vi "Get Status.vi"(6 "timeout (ms)":i32=5000, 8 "error in":errorcluster, 11 "gRPC ID":T10) -> (0 "error out":errorcluster, 2 "Node Status":T1 {"Monitor Doubles"."4" format="%#_9g"; "Monitor Doubles"."3" format="%#_9g"; "Monitor Doubles"."2" format="%#_9g"; "Monitor Doubles"."1" format="%#_9g"}, 3 "gRPC ID out":T10)   [LabVIEW 2021, in "CoreGrpcClientWrapper.lvlib"]
uses:
  CoreGrpcClientWrapper.lvlib
  <vilib>/gRPC/LabVIEW gRPC Library/Shared/grpcId.ctl
  CIFTemplateCommon/Typedef/Plugin Status.ctl
  CIFTemplateCommon/Typedef/Plugin State.ctl
  CIFTemplateCommon/Typedef/Timing Statistics.ctl
  CIFTemplateCommon/Typedef/Timing Stats Base.ctl
  CIFTemplateCommon/Typedef/FIFO Statistics.ctl
  CIFTemplateCommon/Typedef/Simple Error.ctl
  CIFTemplateCommon/Typedef/Monitor Doubles.ctl
  CIFTemplateCommon/Typedef/Monitor U64.ctl
  CIFTemplateCommon/Typedef/Monitor I64.ctl
  CIF_Plugin_Core_client/CIF_Plugin_Core_client.lvlib
  CIFTemplateCommon/CIFTemplateCommon.lvlib
  <vilib>/gRPC/LabVIEW gRPC Library/grpc-lvsupport-release.lvlib
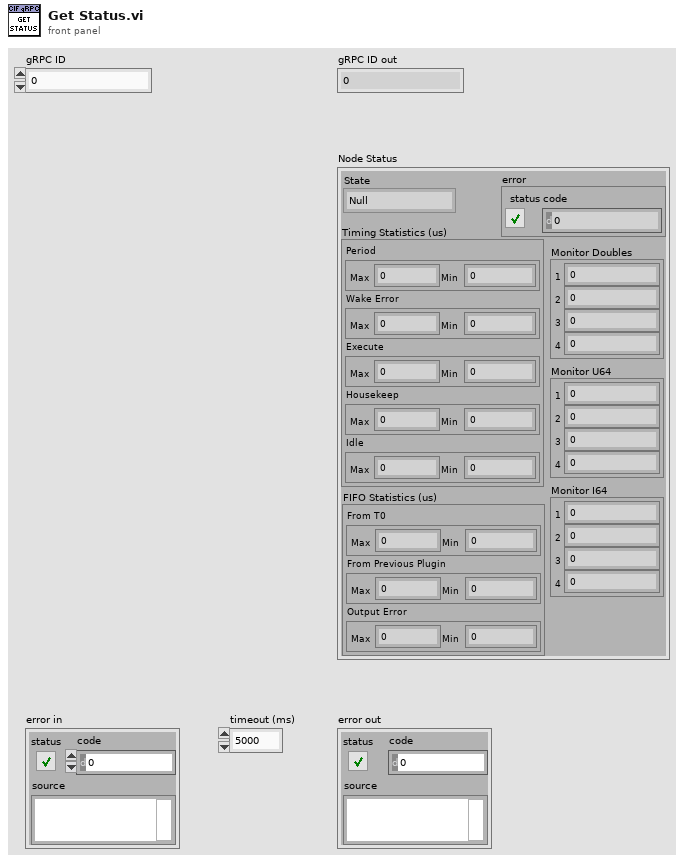
[diagram p1: front panel]
types:
  T1 = typedef "CIFTemplateCommon.lvlib/Plugin Status.ctl" = cluster{"State":T2, "Timing Statistics (us)":T3, "FIFO Statistics (us)":T5, "error":T6, "Monitor Doubles":T7, "Monitor U64":T8, "Monitor I64":T9}
  T2 = typedef "CIFTemplateCommon.lvlib/Plugin State.ctl" = enum32{"Null", "Creating", "Listening", "Running", "CleaningUp", "Destroying"}
  T3 = typedef "CIFTemplateCommon.lvlib/Timing Statistics.ctl" = cluster{"Period":T4, "Wake Error":T4, "Execute":T4, "Housekeep":T4, "Idle":T4}
  T4 = typedef "CIFTemplateCommon.lvlib/Timing Stats Base.ctl" = cluster{"Max":i32, "Min":i32}
  T5 = typedef "CIFTemplateCommon.lvlib/FIFO Statistics.ctl" = cluster{"From T0":T4, "From Previous Plugin":T4, "Output Error":T4}
  T6 = typedef "CIFTemplateCommon.lvlib/Simple Error.ctl" = cluster{"status":bool, "code":i32}
  T7 = typedef "CIFTemplateCommon.lvlib/Monitor Doubles.ctl" = cluster{"1":dbl, "2":dbl, "3":dbl, "4":dbl}
  T8 = typedef "CIFTemplateCommon.lvlib/Monitor U64.ctl" = cluster{"1":u64, "2":u64, "3":u64, "4":u64}
  T9 = typedef "CIFTemplateCommon.lvlib/Monitor I64.ctl" = cluster{"1":i64, "2":i64, "3":i64, "4":i64}
  T10 = typedef "grpc-lvsupport-release.lvlib/grpcId.ctl" = u64
  T11 = typedef "CIF_Plugin_Core_client.lvlib/cif_plugincore_StatusData.ctl" = cluster{"state":T12, "timing_statistics":T13, "fifo_statistics":T15, "error":T16, "monitor_doubles":T17, "monitor_u64s":T18, "monitor_i64s":T19}
  T12 = typedef "CIF_Plugin_Core_client.lvlib/cif_plugincore_StatusData_State.ctl" = enum32{"NULL", "CREATING", "LISTENING", "RUNNING", "CLEANINGUP", "DESTROYING"}
  T13 = typedef "CIF_Plugin_Core_client.lvlib/cif_plugincore_TimingStatistics.ctl" = cluster{"period":T14, "wake_error":T14, "execute":T14, "housekeep":T14, "idle":T14}
  T14 = typedef "CIF_Plugin_Core_client.lvlib/cif_plugincore_TimingStatsBasic.ctl" = cluster{"max":i32, "min":i32}
  T15 = typedef "CIF_Plugin_Core_client.lvlib/cif_plugincore_FifoStatistics.ctl" = cluster{"from_t0":T14, "from_previous_plugin":T14, "output_error":T14}
  T16 = typedef "CIF_Plugin_Core_client.lvlib/cif_plugincore_Error.ctl" = cluster{"status":bool, "code":i32}
  T17 = typedef "CIF_Plugin_Core_client.lvlib/cif_plugincore_MonitorDoubles.ctl" = cluster{"double_1":dbl, "double_2":dbl, "double_3":dbl, "double_4":dbl}
  T18 = typedef "CIF_Plugin_Core_client.lvlib/cif_plugincore_MonitorU64.ctl" = cluster{"u64_1":u64, "u64_2":u64, "u64_3":u64, "u64_4":u64}
  T19 = typedef "CIF_Plugin_Core_client.lvlib/cif_plugincore_MonitorI64.ctl" = cluster{"i64_1":i64, "i64_2":i64, "i64_3":i64, "i64_4":i64}
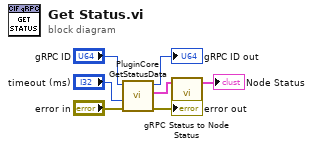
[diagram p0: block diagram]
diagram:
  n1 = call "PluginCore GetStatusData.vi"("error in"="error in", "timeout (ms)"="timeout (ms)", "gRPC ID"="gRPC ID") -> ("error out"=→"error out":errorcluster, "Response Data"=w2:T11, "gRPC ID out"=→"gRPC ID out":T10)  [unwired: 6 in]
  n2 = call "gRPC Status to Node Status.vi"("gRPC Status"=w2) -> ("Node Status"=→"Node Status":T1)  [unwired: 3 in]
